vi "ReportConfiguration.vi"(9 "Destination":T2={"Subsystem Id"=42.0, "Node Id"=1.0, "Component Id"=1.0}, 10 "Source":T2={"Subsystem Id"=90.0, "Node Id"=1.0, "Component Id"=1.0}) -> (2 "Encoded JAUS Message":string)   [LabVIEW 2009]
panel:
  in  "NodeList":T1(array[cluster])=[{"Node Id"=1, "ComponentSeq"=[{"Component Id"=1, "Instance Id"=0}, {"Component Id"=1, "Instance Id"=0}]}]
  in  "Command Code":string="K\u0001"
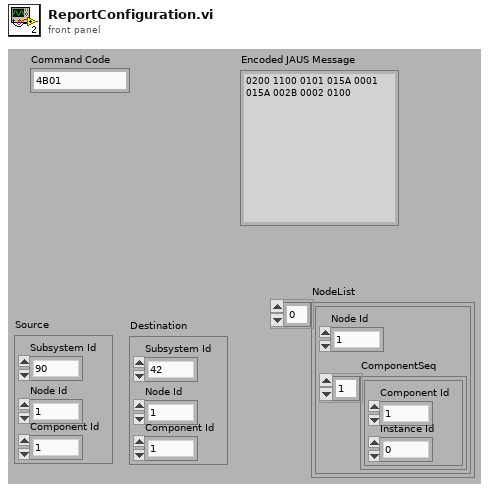
[diagram p1: front panel]
types:
  T1 = cluster{"Node Id":u8, "ComponentSeq":cluster{"Component Id":u8, "Instance Id":u8}[]}[]
  T2 = cluster{"Subsystem Id":dbl, "Node Id":dbl, "Component Id":dbl}
  T3 = cluster{"unsigned byte array[0]":u8, "unsigned byte array[1]":u8}
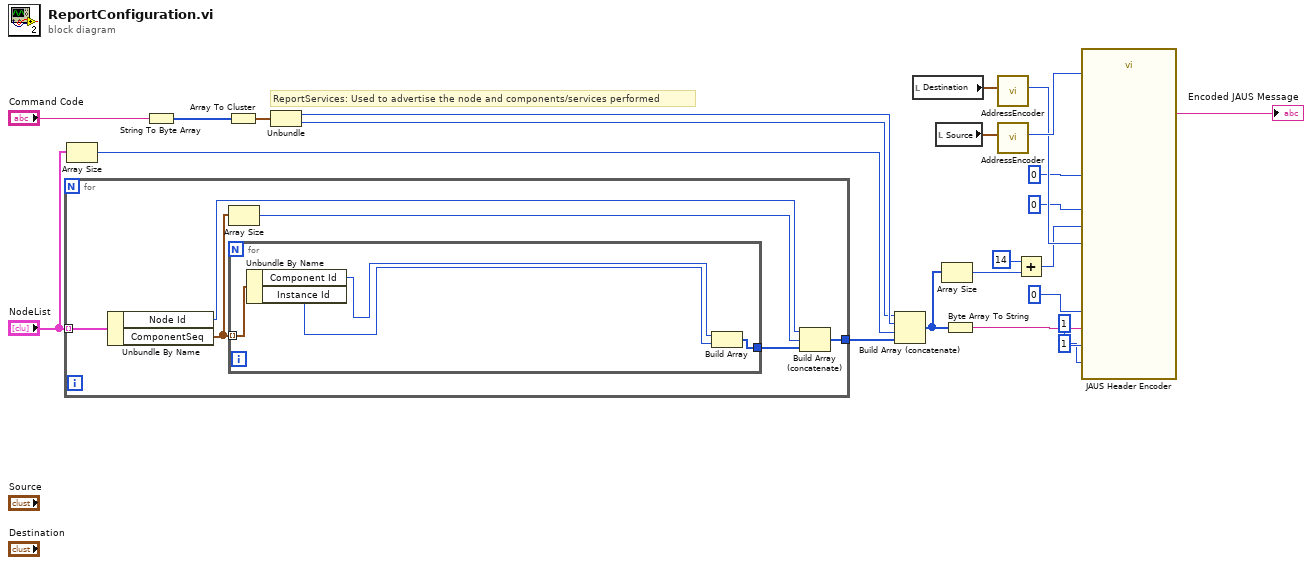
[diagram p0: block diagram]
diagram:
  # "ReportServices: Used to advertise the node and components/services performed"
  n1 = for {
    tunnel: "NodeList" -> [w29] mode=indexing
    tunnel: [w24] -> w5
    n2 = Unbundle By Name(w29) -> ("Node Id"=w28:u8, "ComponentSeq"=w27:cluster{"Component Id":u8, "Instance Id":u8}[])
    n3 = Array Size(array=w27) -> (size(s)=w26:i32)
    n4 = for {
      tunnel: w27 -> [w32] mode=indexing
      tunnel: [w33] -> w25
      n5 = Unbundle By Name(w32) -> ("Component Id"=w31:u8, "Instance Id"=w30:u8)
      n6 = Build Array(w31, w30) -> (w33:u8[])
    }
    n7 = Build Array (concatenate)(w28, w26, w25) -> (w24:i32[])
  }
  n8 = Array Size(array="NodeList") -> (size(s)=w7:i32)
  n9 = String To Byte Array(string="Command Code") -> (unsigned byte array=w11:u8[])
  n10 = Array To Cluster(array=w11) -> (cluster=w10:T3)
  n11 = Unbundle(w10) -> ("unsigned byte array[0]"=w9:u8, "unsigned byte array[1]"=w8:u8)
  n12 = Build Array (concatenate)(w8, w9, w7, w5) -> (w4:i32[])
  n13 = local read "Destination"() -> (w20:T2)
  n14 = local read "Source"() -> (w22:T2)
  n15 = Array Size(array=w4) -> (size(s)=w2:i32)
  n16 = Byte Array To String(unsigned byte array=w4) -> (string=w13:string)
  n17 = call "AddressEncoder.vi"("Address Cluster"=w20) -> ("Address"=w19:u32)  [unwired: 10 in]
  n18 = call "AddressEncoder.vi"("Address Cluster"=w22) -> ("Address"=w21:u32)  [unwired: 10 in]
  n19 = Add(x=u8 14 ("Data Size (8-23)"), y=w2) -> (x+y=w1:i32)
  n20 = call "JAUS Header Encoder.vi"("Message Type (0-5)"=u8 0, "Data Size (8-23)"=w1, "Priority(40-41)"=u8 1, "Sequence Number (16 bits)"=u16 1, "Payload"=w13, "Source ID (80-95)"=w21, "Destination ID (48-79)"=w19, "Data Flags (46-47)"=u8 0, "Ack/Nak (44-45)"=u8 0) -> ("Encoded JAUS Message"=→"Encoded JAUS Message":string)  [unwired: 6 in]
